vi "ConstantToArray_U64Rgba.vi"(11 "Rgba":T1) -> (3 "ConstantArray":dbl[](array[numeric]))   [LabVIEW 2020, in "OpenLvVision_OpenCv.lvlib"]
uses:
  OpenLvVision_OpenCv.lvlib
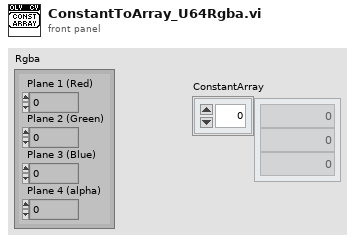
[diagram p1: front panel]
types:
  T1 = typedef "Color (U64)" = cluster{"Plane 3 (Blue)":u16, "Plane 2 (Green)":u16, "Plane 1 (Red)":u16, "Plane 4 (alpha)":u16}
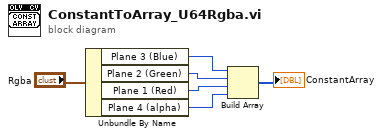
[diagram p0: block diagram]
diagram:
  n1 = Unbundle By Name("Rgba") -> ("Plane 3 (Blue)"=w6:u16, "Plane 2 (Green)"=w5:u16, "Plane 1 (Red)"=w4:u16, "Plane 4 (alpha)"=w3:u16)
  n2 = Build Array(w6, w5, w4, w3) -> (→"ConstantArray":u16[])
